vi "Untitled 1.vi"() -> ()   [LabVIEW 2020]
uses:
  <vilib>/Instr/_visa.llb/VISA Configure Serial Port (Instr).vi
  <vilib>/Utility/file.llb/Write Delimited Spreadsheet (string).vi
panel:
  in  "开关":bool=TRUE
  in  "文件\n路径":path=path "C:/Users/Lenovo/Desktop/data.xls"
  out "错误输出":cluster{"status":bool, i32, string}={"status"=FALSE, 1073676294, "VISA Read in Untitled 1.vi"}
  out "D2  逻辑值":dbl
  out "?":cluster{i32, i32}(graph)={31, 61}
  in  "字节数(5)":u32=5
  out "缓存区":string="23161"
  in  "串口":refnum<visa-resource-name>="COM4"
  in  "等待时间(ms)":u32=200
  in  "串口设置":T1={"流控制 (0:none)"=0, "停止位 (10: 1 bit)"=10, "奇偶校验 (0:none)"=0, "数据比特 (8)"=8, "比特率 (115200)"=115200} {"数据比特 (8)" min=5 max=8 step=1; "奇偶校验 (0:none)" items=["None", "Odd", "Even", "Mark", "Space"]; "流控制 (0:none)" items=["None", "XON/XOFF", "RTS/CTS", "XON/XOFF & RTS/CTS", "DTR/DSR", "XON/XOFF & DTR/DSR"]}
  out "湿度":i32=61
  out "温度":i32=31
  # "数据"
  # "基于LabView和单片机的温湿度实时监测网络平台系统"
  # "安徽大学集成光电器件工程训练"
  # "指导教师:李劲松"
  # "B01914005 苏柯宁"
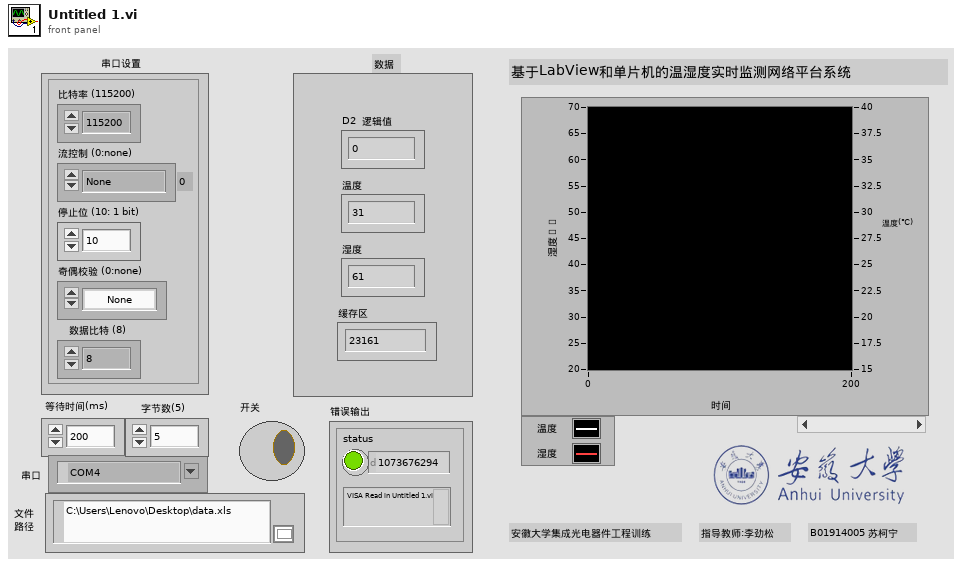
[diagram p1: front panel]
types:
  T1 = cluster{"流控制 (0:none)":u16, "停止位 (10: 1 bit)":u16, "奇偶校验 (0:none)":u16, "数据比特 (8)":u16, "比特率 (115200)":u32}
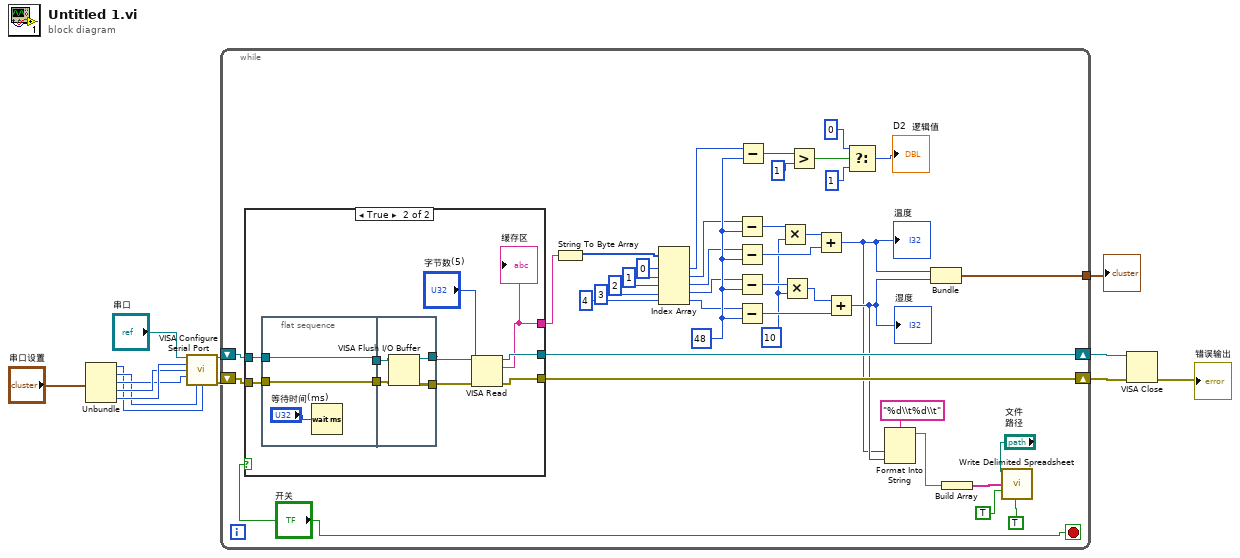
[diagram p0: block diagram]
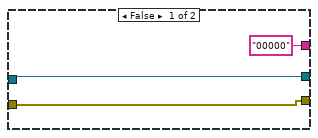
[diagram p2: hidden frame]
diagram:
  n1 = Unbundle("串口设置") -> ("流控制 (0:none)"=w5:u16, "停止位 (10: 1 bit)"=w6:u16, "奇偶校验 (0:none)"=w7:u16, "数据比特 (8)"=w8:u16, "比特率 (115200)"=w9:u32)
  n2 = call-poly "VISA Configure Serial Port"("VISA resource name"="串口", "baud rate (9600)"=w9, "data bits (8)"=w8, "parity (0:none)"=w7, "stop bits (10: 1 bit)"=w6, "flow control (0:none)"=w5) -> ("VISA resource name out"=w13:refnum<visa-resource-name>, "error out"=w12:errorcluster)  [unwired: 8 in]
  n3 = while {
    shift-right: [w50] -> w3
    shift-left: w13 -> [w53]
    shift-right: [w51] -> w4
    shift-left: w12 -> [w52]
    tunnel: [w14] -> w1
    stop <- "开关" stop-if-true
    w32 = 10 ("y")
    w44 = 48
    n4 = case shown="True" "开关" {
      tunnel: w53 -> [w56 w64]
      tunnel: w52 -> [w55 w63]
      tunnel: [w55 w62] -> w51
      tunnel: [w56 w61] -> w50
      tunnel: ["00000" ("read buffer") w57] -> w17
      frame False {
      }
      frame True {
        n5 = flat-sequence {
          tunnel: [w69] -> w66
          tunnel: w64 -> [w69]
          tunnel: w63 -> [w68]
          tunnel: [w68] -> w65
          tunnel: [w73] -> w59
          tunnel: w66 -> [w72]
          tunnel: w65 -> [w71]
          tunnel: [w70] -> w60
          frame #0 {
            n6 = Wait (ms)(milliseconds to wait="等待时间(ms)") -> ()  [unwired: 1 out]
          }
          frame #1 {
            n7 = VISA Flush I/O Buffer(VISA resource name=w72, error in (no error)=w71) -> (VISA resource name out=w73:refnum<visa-resource-name>, error out=w70:errorcluster)  [unwired: 1 in]
          }
        }
        n8 = VISA Read(VISA resource name=w59, byte count="字节数(5)", error in (no error)=w60) -> (VISA resource name out=w61:refnum<visa-resource-name>, read buffer=w57:string, error out=w62:errorcluster)  [unwired: 1 out]
        "缓存区" <- w57
      }
    }
    n9 = String To Byte Array(string=w17) -> (unsigned byte array=w16:u8[])
    n10 = Index Array(array=w16, index #1=0 ("index"), index #2=1 ("index"), index #3=2 ("index"), index #4=3 ("index"), index #5=4 ("index")) -> (element #1=w43:u8, element #2=w42:u8, element #3=w41:u8, element #4=w40:u8, element #5=w39:u8)
    n11 = Subtract(x=w42, y=w44) -> (x-y=w38:i32)
    n12 = Subtract(x=w41, y=w44) -> (x-y=w36:i32)
    n13 = Subtract(x=w40, y=w44) -> (x-y=w35:i32)
    n14 = Subtract(x=w39, y=w44) -> (x-y=w33:i32)
    n15 = Subtract(x=w43, y=w44) -> (x-y=w31:i32)
    n16 = Multiply(x=w38, y=w32) -> (x*y=w37:i32)
    n17 = Multiply(x=w35, y=w32) -> (x*y=w34:i32)
    n18 = Greater?(x=w31, y=1) -> (0:w29:bool)
    n19 = Add(x=w37, y=w36) -> (x+y=w20:i32)
    "温度" <- w20
    n20 = Add(x=w34, y=w33) -> (x+y=w25:i32)
    "湿度" <- w25
    n21 = Select(t=i16 0, s=w29, f=i16 1) -> (s? t:f=→"D2  逻辑值":i16)
    n22 = Format Into String(format string="%d\\t%d\\t", w20, w25) -> (resulting string=w24:string)  [unwired: 2 in, 1 out]
    n23 = Bundle(w20, w25) -> (w14:cluster{i32, i32})  [unwired: 1 in]
    n24 = Build Array(w24) -> (w23:string[])
    n25 = call-poly <vilib>:"Write Delimited Spreadsheet.vi"("file path (dialog if empty)"="文件\n路径", "1D data"=w23, "append to file? (new file:F)"=TRUE, "transpose? (no:F)"=TRUE) -> ()  [unwired: 10 in, 2 out]
  }
  "?" <- w1
  n26 = VISA Close(VISA resource name=w3, error in (no error)=w4) -> (error out=→"错误输出":errorcluster)
